vi "VIinClass.vi"(9 "Y":dbl, 10 "X":dbl) -> (3 "Result":dbl)   [LabVIEW 2023, in "ClassForClassMemberCall.lvclass"]
uses:
  ClassForClassMemberCall.lvclass
  ClassForClassMemberCall.lvclass/ClassForClassMemberCall.ctl
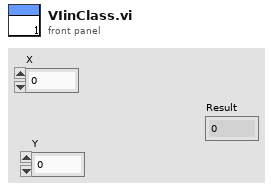
[diagram p1: front panel]
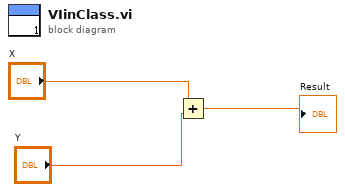
[diagram p0: block diagram]
diagram:
  n1 = Add(x="X", y="Y") -> (x+y=→"Result":dbl)
